vi "Write JSON.vi"(8 "error in (no error)":errorcluster, 10 "JSON":string="{}", 11 "CycloneDX JSON in":refnum<class "CycloneDX JSON.lvclass">) -> (0 "error out":errorcluster, 3 "CycloneDX JSON out":refnum<class "CycloneDX JSON.lvclass">)   [LabVIEW 2017, in "LabVIEW CycloneDX SBOM.lvlib" / "CycloneDX JSON.lvclass"]
uses:
  CycloneDX JSON.lvclass
  CycloneDX JSON.lvclass/CycloneDX JSON.ctl
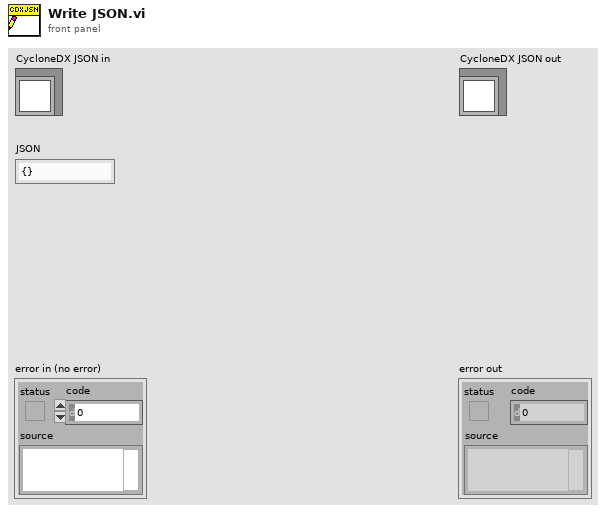
[diagram p1: front panel]
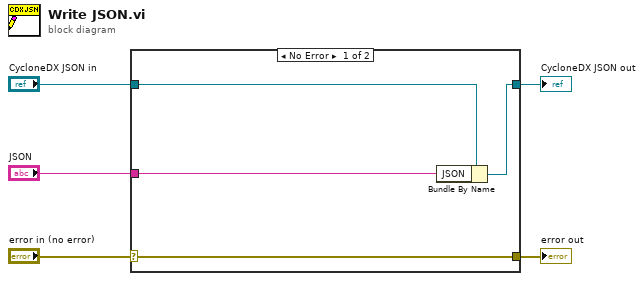
[diagram p0: block diagram]
diagram:
  n1 = case shown="No Error" "error in (no error)" {
    selector: "error in (no error)" -> [w9 w10]
    tunnel: [w9 w10] -> w4
    tunnel: [w7 w11] -> w2
    tunnel: "CycloneDX JSON in" -> [w8 w11]
    tunnel: "JSON" -> [w6 _]
    frame No Error {
      n2 = Bundle By Name(cluster=w8, "JSON"=w6) -> (w7:refnum<class "CycloneDX JSON.lvclass">)
    }
    frame Error {
    }
  }
  "error out" <- w4
  "CycloneDX JSON out" <- w2
